vi "MSGR Object Modify.vi"(7 "function":enum16{"set data", "function 1", "modify data"}(ring)=enum."function 1", 8 "error in (no error)":errorcluster, 9 "destroy (F)":bool, 10 "parameter":dbl format="%.2f", 11 "object":T1) -> (0 "error out":errorcluster, 2 "parameter out":dbl format="%.2f", 3 "object out":T1)   [LabVIEW 2018]
doc: "$Author::Richard Jennings $\n$Rev:: $\n$Date:: May, 2008 $\n\nOVERVIEW:\nReentrant VI to receive messages via a MSGR Q. If the Q does not exist this VI will create it, then wait for data.\n\nINPUTS (Controls):\n<name> - <short description of each control wired to connector pane>\n\nOUTPUTS (Indicators):\n<name> - <short description of each indicator wired to connector pane>\n\nCopyright 2008 - 2017 Jennings Embedded Servies. All rights reserved.\nAuthor makes no warranties or guarantees related to performance of the software.\nUSE AT YOUR OWN RISK\nwww.jembedded.com\n\n\n\nMIT License\n\nCopyright (c) 2020 RichardLGP5\n\nPermission is hereby granted, free of charge, to any person obtaining a copy\nof this software and associated documentation files (the \"Software\"), to deal\nin the Software without restriction, including without limitation the rights\nto use, copy, modify, merge, publish, distribute, sublicense, and/or sell\ncopies of the Software, and to permit persons to whom the Software is\nfurnished to do so, subject to the following conditions:\n\nThe above copyright notice and this permission notice shall be included in all\ncopies or substantial portions of the Software.\n\nTHE SOFTWARE IS PROVIDED \"AS IS\", WITHOUT WARRANTY OF ANY KIND, EXPRESS OR\nIMPLIED, INCLUDING BUT NOT LIMITED TO THE WARRANTIES OF MERCHANTABILITY,\nFITNESS FOR A PARTICULAR PURPOSE AND NONINFRINGEMENT. IN NO EVENT SHALL THE\nAUTHORS OR COPYRIGHT HOLDERS BE LIABLE FOR ANY CLAIM, DAMAGES OR OTHER\nLIABILITY, WHETHER IN AN ACTION OF CONTRACT, TORT OR OTHERWISE, ARISING FROM,\nOUT OF OR IN CONNECTION WITH THE SOFTWARE OR THE USE OR OTHER DEALINGS IN THE\nSOFTWARE."
uses:
  MSGR Registry Control TypeDef.ctl
  Object.ctl
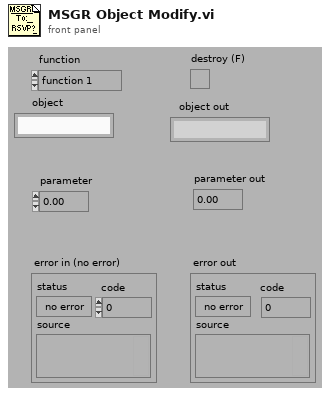
[diagram p1: front panel]
types:
  T1 = typedef "Object.ctl" = string
  T2 = typedef "MSGR Registry Control TypeDef.ctl" = enum16{"reset", "register", "get data", "set data", "unregister", "test", "get objects"}
  T3 = typedef "MSGR Q Ref TypeDef.ctl" = refnum<queue>
  T4 = typedef "MSGR Q Name TypeDef.ctl" = string
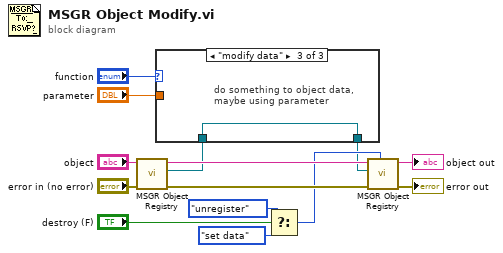
[diagram p0: block diagram]
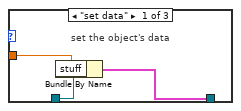
[diagram p2: hidden frame]
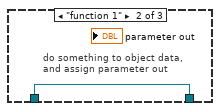
[diagram p3: hidden frame]
diagram:
  n1 = call "MSGR Object Registry.vi"("error in (no error)"="error in (no error)", "MSGR Q name"="object") -> ("error out"=w13:errorcluster, "MSGR Q"=w7:T3, "MSGR Q name"=w10:T4)  [unwired: 5 in, 2 out]
  n2 = case shown="\"modify data\"" "function" {
    tunnel: w7 -> [w16 w18 w19]
    tunnel: [w17 w18 w19] -> w1
    tunnel: "parameter" -> [w15 _ _]
    frame "set data" {
      # "set the object's data"
      n3 = Bundle By Name(cluster=w16, "stuff"=w15) -> (w17:cluster{})
    }
    frame "function 1" {
      # "do something to object data,\nand assign parameter out"
    }
    frame "modify data" {
      # "do something to object data,\nmaybe using parameter"
    }
  }
  n4 = Select(t=MSGR_Registry_Control_TypeDef."unregister" ("function (get data)"), s="destroy (F)", f=MSGR_Registry_Control_TypeDef."set data" ("function (get data)")) -> (s? t:f=w2:T2)
  n5 = call "MSGR Object Registry.vi"("function (get data)"=w2, "error in (no error)"=w13, "MSGR Q"=w1, "MSGR Q name"=w10) -> ("error out"=→"error out":errorcluster, "MSGR Q name"=→"object out":T4)  [unwired: 3 in, 3 out]
